vi "Open Template Class.vi"(8 "error in (no error)":errorcluster, 11 "Application in":refnum<vi>) -> (0 "error out":errorcluster, 2 "Template Class Methods and Controls":refnum<vi>[](array[refnum]), 3 "Template Class Refnum out":refnum<vi>)   [LabVIEW 2015, in "QControl Creation.lvclass"]
doc: "<b> </b> <b> </b>\n©2016 Q Software Innovations, LLC (QSI)\nwritten by Quentin Alldredge\nproduced in LabVIEW 2015\n\nsupport@qsoftwareinnovations.com\nwww.qsoftwareinnovations.com\n\nAll rights reserved.\n\nRedistribution and use in source and binary forms, with or without modification, are permitted provided that the following conditions are met:\n\n * Redistributions of source code must retain the above copyright notice, this list of conditions and the following disclaimer.\n * Redistributions in binary form must reproduce the above copyright notice, this list of conditions and the following disclaimer in the documentation and/or other materials provided with the distribution.\n * Neither the name of Q Software Innovations, LLC. nor the names of its contributors may be used to endorse or promote products derived from this software without specific prior written permission.\n\nTHIS SOFTWARE IS PROVIDED BY THE COPYRIGHT HOLDERS AND CONTRIBUTORS \"AS IS\" AND ANY EXPRESS OR IMPLIED WARRANTIES, INCLUDING, BUT NOT LIMITED TO, THE IMPLIED WARRANTIES OF MERCHANTABILITY AND FITNESS FOR A PARTICULAR PURPOSE ARE DISCLAIMED. IN NO EVENT SHALL THE COPYRIGHT OWNER OR CONTRIBUTORS BE LIABLE FOR ANY DIRECT, INDIRECT, INCIDENTAL, SPECIAL, EXEMPLARY, OR CONSEQUENTIAL DAMAGES (INCLUDING, BUT NOT LIMITED TO, PROCUREMENT OF SUBSTITUTE GOODS OR SERVICES; LOSS OF USE, DATA, OR PROFITS; OR BUSINESS INTERRUPTION) HOWEVER CAUSED AND ON ANY THEORY OF LIABILITY, WHETHER IN CONTRACT, STRICT LIABILITY, OR TORT (INCLUDING NEGLIGENCE OR OTHERWISE) ARISING IN ANY WAY OUT OF THE USE OF THIS SOFTWARE, EVEN IF ADVISED OF THE POSSIBILITY OF SUCH DAMAGE."
uses:
  QControl Creation.lvclass
  Template/Template.lvclass
  <vilib>/ErrorRing/Error Ring.xnode
  <vilib>/Utility/error.llb/Error Cluster From Error Code.vi
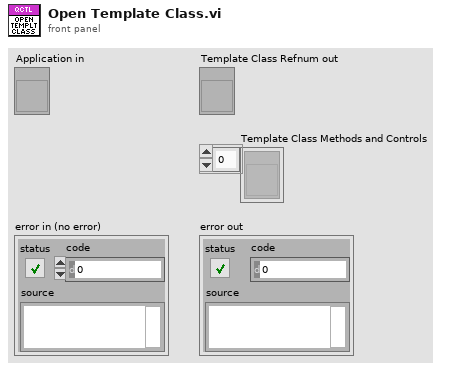
[diagram p1: front panel]
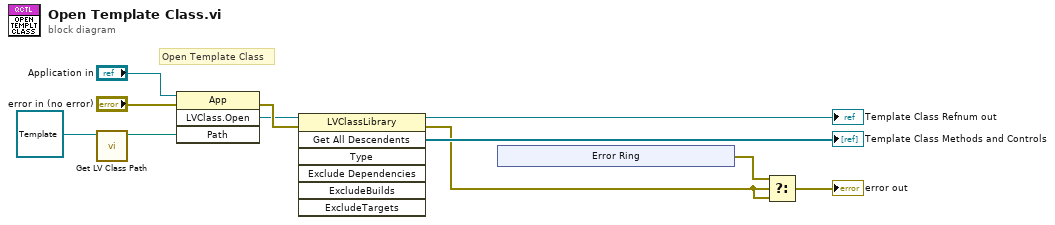
[diagram p0: block diagram]
diagram:
  # "Open Template Class"
  n1 = call <vilib>:"Get LV Class Path.vi"("object"=refnum<class "Template.lvclass"> refnum ("Template")) -> ("class path"=w9:path)  [unwired: 9 in, 1 out]
  n2 = invoke class="App" method="LVClass.Open"(reference="Application in", error in="error in (no error)", "Path"=w9) -> (error out=w5:errorcluster, "LVClass.Open"=w4:refnum<vi>)  [unwired: 1 in, 2 out]
  n3 = invoke class="LVClassLibrary" method="Get All Descendents"(reference=w4, error in=w5) -> (reference out=→"Template Class Refnum out":refnum<vi>, error out=w1:errorcluster, "All Descendents"=→"Template Class Methods and Controls":refnum<vi>[])  [unwired: 5 in, 4 out]
  n4 = xnode "Error Ring"() -> ("error out"=w3:errorcluster)
  n5 = Select(t=w3, s=w1, f=w1) -> (s? t:f=→"error out":errorcluster)
